vi "Autotest_Instr.vi"(8 "error in (no error)":errorcluster caption="entrée d'erreur (pas d'erreur)", 11 "Class Instrument (Default) en entrée":refnum<class "Class Instrument Printer.lvclass">) -> (0 "error out":errorcluster caption="sortie d'erreur", 3 "Class Instrument (Default) en sortie":refnum<class "Class Instrument Printer.lvclass">)   [LabVIEW 2020, in "Library Instrument & Equipement.lvlib" / "Library Instruments.lvlib" / "Class Instrument Printer.lvclass"]
uses:
  Class Instrument Printer.lvclass
  C:/Users/ngarcin/OneDrive - Altyor/Standard TB/Class/Instrument/Instrument (Default)/Class Instrument (Default).lvclass
  Class Instrument Printer.lvclass/Class Instrument Printer.ctl
  Instrument (Default)/Class Instrument (Default).lvclass
  Printer/Printer (Default)/Class Printer (Default).lvclass
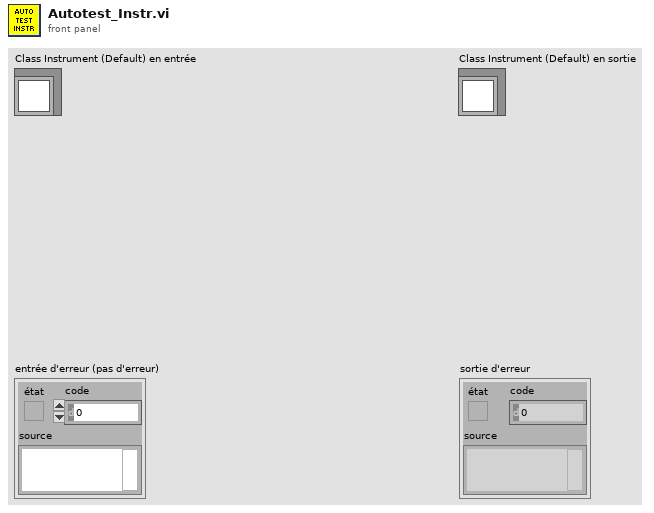
[diagram p1: front panel]
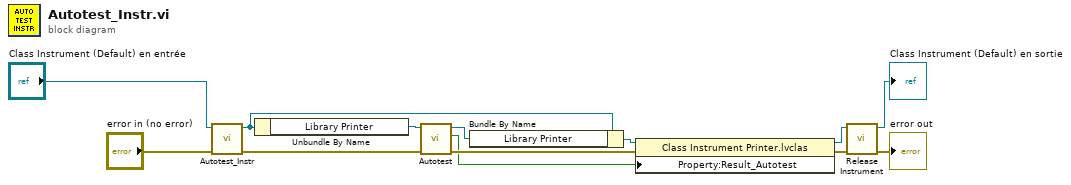
[diagram p0: block diagram]
diagram:
  n1 = call-parent "Autotest_Instr.vi"("error in (no error)"="error in (no error)", "Class Instrument (Default) en entrée"="Class Instrument (Default) en entrée") -> ("error out"=w11:errorcluster, "Class Instrument (Default) en sortie"=w5:refnum<class "Class Instrument Printer.lvclass">)  [unwired: 8 in]
  n2 = Unbundle By Name(w5) -> ("Library Printer"=w10:refnum<class "Class Printer (Default).lvclass">)
  n3 = call-dynamic "Autotest.vi"("error in (no error)"=w11, "Class Printer (Default) en entrée"=w10) -> ("error out"=w6:errorcluster, "Autotest Ok ?"=w1:bool, "Class Printer (Default) en sortie"=w2:refnum<class "Class Printer (Default).lvclass">)  [unwired: 7 in]
  n4 = Bundle By Name(cluster=w5, "Library Printer"=w2) -> (w9:refnum<class "Class Instrument Printer.lvclass">)
  n5 = property class="Class Instrument Printer.lvclas"(reference=w9, error in=w6, "Property:Result_Autotest"=w1) -> (reference out=w7:refnum<class "Class Instrument Printer.lvclass">, error out=w8:errorcluster)
  n6 = call-dynamic "Release Instrument.vi"("error in (no error)"=w8, "Class Instrument (Default) en entrée"=w7) -> ("error out"=→"error out":errorcluster, "Class Instrument (Default) en sortie"=→"Class Instrument (Default) en sortie":refnum<class "Class Instrument Printer.lvclass">)  [unwired: 8 in]
